vi "Stop Core.vi"(10 "final error code":i32, 11 "Async Methods Actor in":refnum<class "Async Methods Actor.lvclass">) -> (3 "Async Methods Actor out":refnum<class "Async Methods Actor.lvclass">)   [LabVIEW 2021, in "Async Methods Actor.lvlib" / "Async Methods Actor.lvclass"]
doc: "(<B>Filename</B>: Actor Framework.lvlib:Actor.lvclass:Stop Core.vi)\n\nDefines what the actor does before it stops. Use the <B>final error code</B> input to determine whether the actor shut down in response to an error.\n\nBy default, this method passes the Stop message along to all auto-stop nested actors. A descendant class may override this method to define additional behavior, such as shutting down any processes the actor initiated in its override of the Actor Core method."
uses:
  Async Methods Actor.lvclass
  Async Methods Actor.lvclass/Async Methods Actor.ctl
  08967ba7-e6e7-44cc-a44e-d91714aa85c9.vi
  cebc0adc-4ac4-48a5-9627-4995084fc216.vi
  <vilib>/ActorFramework/Actor/Actor.lvclass
  Async Methods Actor Messages/Async Message/Async Message.lvclass
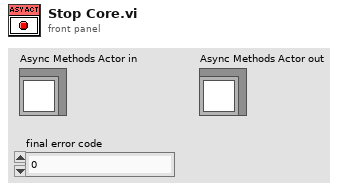
[diagram p1: front panel]
types:
  T1 = typedef "Async Methods Actor.lvlib/Async Methods Actor.lvclass/VI Refnums Map.ctl" = map{refnum<vi>, T2}
  T2 = typedef "Async Methods Actor.lvlib/Async Methods Actor.lvclass/VI Refnums Map Value.ctl" = cluster{"Async Call Method":T3, "VI Refnum Lifecycle":T4, "Message Path":path}
  T3 = typedef "Async Methods Actor.lvlib/Async Methods Actor.lvclass/Async Call Method.ctl" = enum16{"Call and Collect", "Call and Forget"}
  T4 = typedef "Async Methods Actor.lvlib/Async Methods Actor.lvclass/VI Refnum Lifetime.ctl" = enum16{"Destroy on Exit", "Destroy on Actor Exit", "Leak"}
  T5 = typedef "Async Methods Actor.lvlib/Async Methods Actor.lvclass/Running Methods Communication.ctl" = enum16{"None", "Notifier", "Event"}
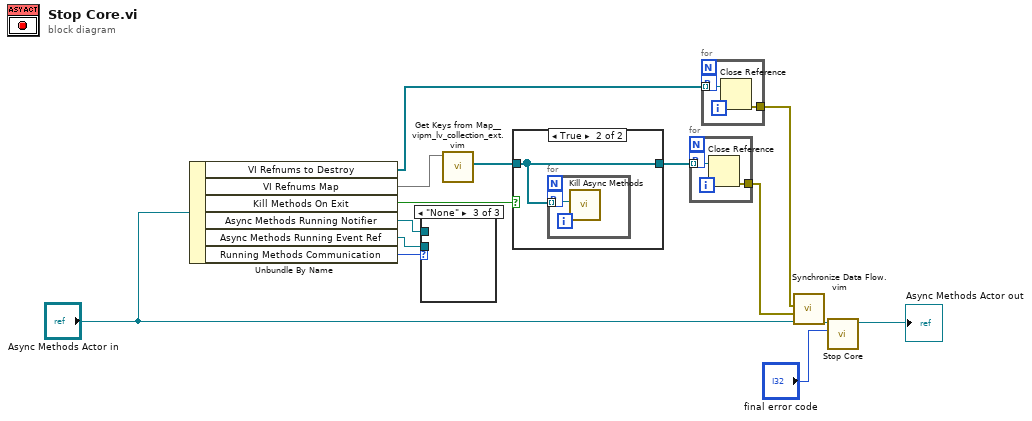
[diagram p0: block diagram]
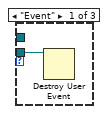
[diagram p2: hidden frame]
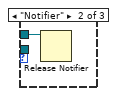
[diagram p3: hidden frame]
diagram:
  n1 = Unbundle By Name("Async Methods Actor in") -> ("VI Refnums to Destroy"=w2:refnum<vi>[], "VI Refnums Map"=w13:T1, "Kill Methods On Exit"=w12:bool, "Async Methods Running Notifier"=w8:refnum<notifier>, "Async Methods Running Event Ref"=w3:refnum<user-event>, "Running Methods Communication"=w4:T5)
  n2 = case shown="\"None\"" w4 {
    tunnel: w8 -> [_ w16 _]
    tunnel: w3 -> [w15 _ _]
    frame "Event" {
      n3 = Destroy User Event(user event=w15) -> ()  [unwired: 1 in, 1 out]
    }
    frame "Notifier" {
      n4 = Release Notifier(notifier=w16) -> ()  [unwired: 2 in, 3 out]
    }
    frame "None" {
    }
  }
  n5 = call "Get Keys from Map__vipm_lv_collection_ext.vim"("map"=w13) -> ("keys"=w10:refnum<vi>[])  [unwired: 9 in, 1 out]
  n6 = case shown="True" w12 {
    tunnel: w10 -> [w17 w18]
    tunnel: [w17 w18] -> w9
    frame False {
    }
    frame True {
      n7 = for {
        tunnel: w18 -> [w19] mode=indexing
        workers-P: _ -> [_]
        n8 = call "Kill Async Methods.vi"("VI Refnum"=w19) -> ()  [unwired: 10 in, 1 out]
      }
    }
  }
  n9 = for {
    tunnel: w9 -> [w21] mode=indexing
    tunnel: [w20] -> w7
    workers-P: _ -> [_]
    n10 = Close Reference(reference=w21) -> (error out=w20:errorcluster)  [unwired: 1 in]
  }
  n11 = for {
    tunnel: w2 -> [w23] mode=indexing
    tunnel: [w22] -> w1
    workers-P: _ -> [_]
    n12 = Close Reference(reference=w23) -> (error out=w22:errorcluster)  [unwired: 1 in]
  }
  n13 = call "Synchronize Data Flow.vim"("input 4"="Async Methods Actor in", "input 3"=w7, "input 2"=w1) -> ("output 4"=w11:refnum<class "Async Methods Actor.lvclass">)  [unwired: 1 in, 3 out]
  n14 = call-parent "Stop Core.vi"("final error code"="final error code", "Actor in"=w11) -> ("Actor out"=→"Async Methods Actor out":refnum<class "Async Methods Actor.lvclass">)  [unwired: 9 in]
